vi "Illini Hyperloop GUI v2.vi"() -> ()   [LabVIEW 2015]
uses:
  <vilib>/robotics/Controls/Attitude Indicator/Attitude Indicator.xctl
  <vilib>/ErrorRing/Error Ring.xnode
panel:
  out "Attitude Indicator":cluster{"Roll":dbl, "Pitch":dbl}(xcontrol)
  out "Yaw":dbl(knob) scale=-90.0..90.0
  out "CO2 Levels":dbl format="%#.3g%%"
  out "O2 Levels":dbl format="%#.3g%%"
  out "Temperature 2":dbl(slide) scale=0.0..400.0
  out "Temp 2:":dbl format="%.2g"
  out "Temp 1:":dbl format="%.2g"
  out "Temperature 1":dbl(slide) scale=0.0..400.0
  out "Cabin Pressure":dbl format="%#.3g"
  out "Pressure":dbl(slide) scale=0.0..20.0
  out "Battery 3:":dbl format="%#.2g"
  out "Battery 2:":dbl format="%#.2g"
  out "Battery 1:":dbl format="%#.2g"
  out "Battery 3":dbl(slide) scale=0.0..100.0
  out "Battery 2":dbl(slide) scale=0.0..100.0
  out "Battery 1":dbl(slide) scale=0.0..100.0
  out "Z acceleration":dbl
  out "Y acceleration":dbl
  out "X acceleration":dbl
  out "Z velocity":dbl
  out "Y velocity":dbl
  out "X velocity":dbl
  out "Z position":dbl
  out "Y position":dbl
  out "X position":dbl
  out "Position (m)":dbl(slide) scale=0.0..2490.0
  in  "EMERGENCY STOP":bool
  out "Data out":string
  in  "Client Closed":string="The client VI closed the connection."
  in  "Functional Test 1":bool caption="Boolean"
  in  "Functional Test 2":bool caption="Boolean"
  in  "Functional Test 4":bool caption="Boolean"
  in  "Functional Test 3":bool caption="Boolean"
  out "Alarms":dbl
  out "Enum":enum16{"All Systems Nominal", "Alarm", ""}(ring)
  out "Ring":u16(ring)
  out "Velocity (m/s)":dbl(graph)
  out "Position":dbl
  out "Velocity":dbl
  out "Acceleration":dbl
  # "Illini Hyperloop"
  # "Functional Test A"
  # "Power Up"
  # "All Systems"
  # "*RESULTS DISPLAYED HERE*"
  # "Acceleration (m/s/s)"
  # "Functional Test B"
  # "Levitation"
  # "*RESULTS DISPLAYED HERE*"
  # "Functional Test C"
  # "Communication"
  # "Battery Levels (%)"
  # "Cabin Pressure (psi)"
  # "O2 Level"
  # "*RESULTS DISPLAYED HERE*"
  # "CO2 Level"
  # "Functional Test D"
  # "Internal Power"
  # "Attitude"
  # "*RESULTS DISPLAYED HERE*"
  # "Temperature (K)"
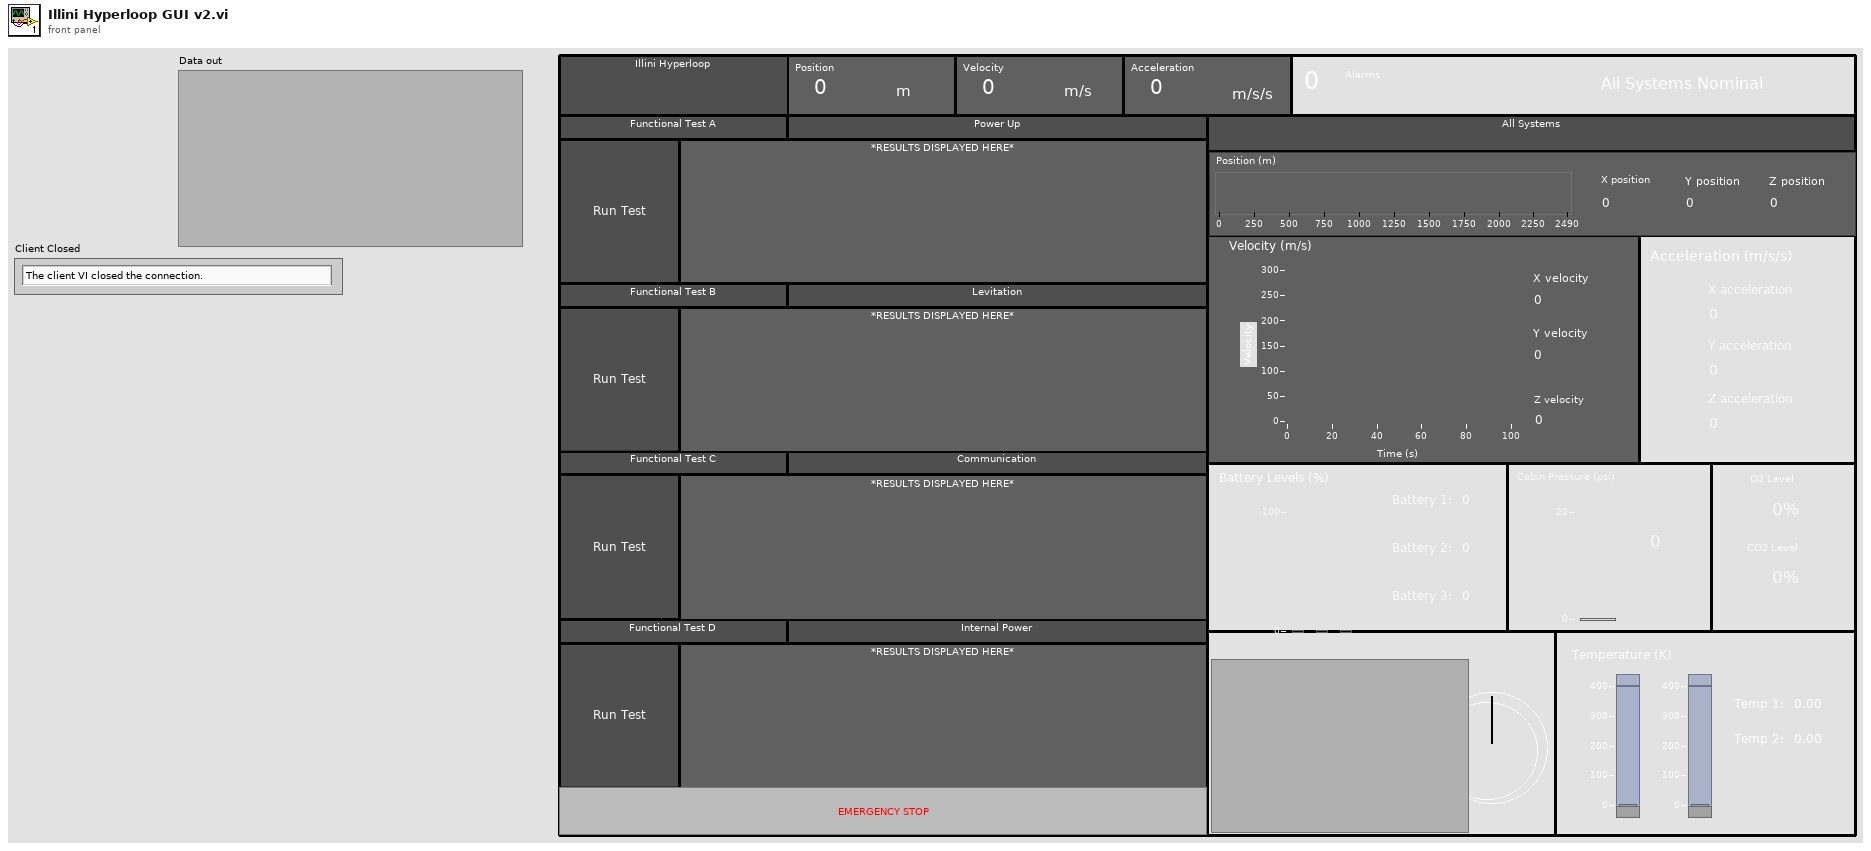
[diagram p1: front panel]
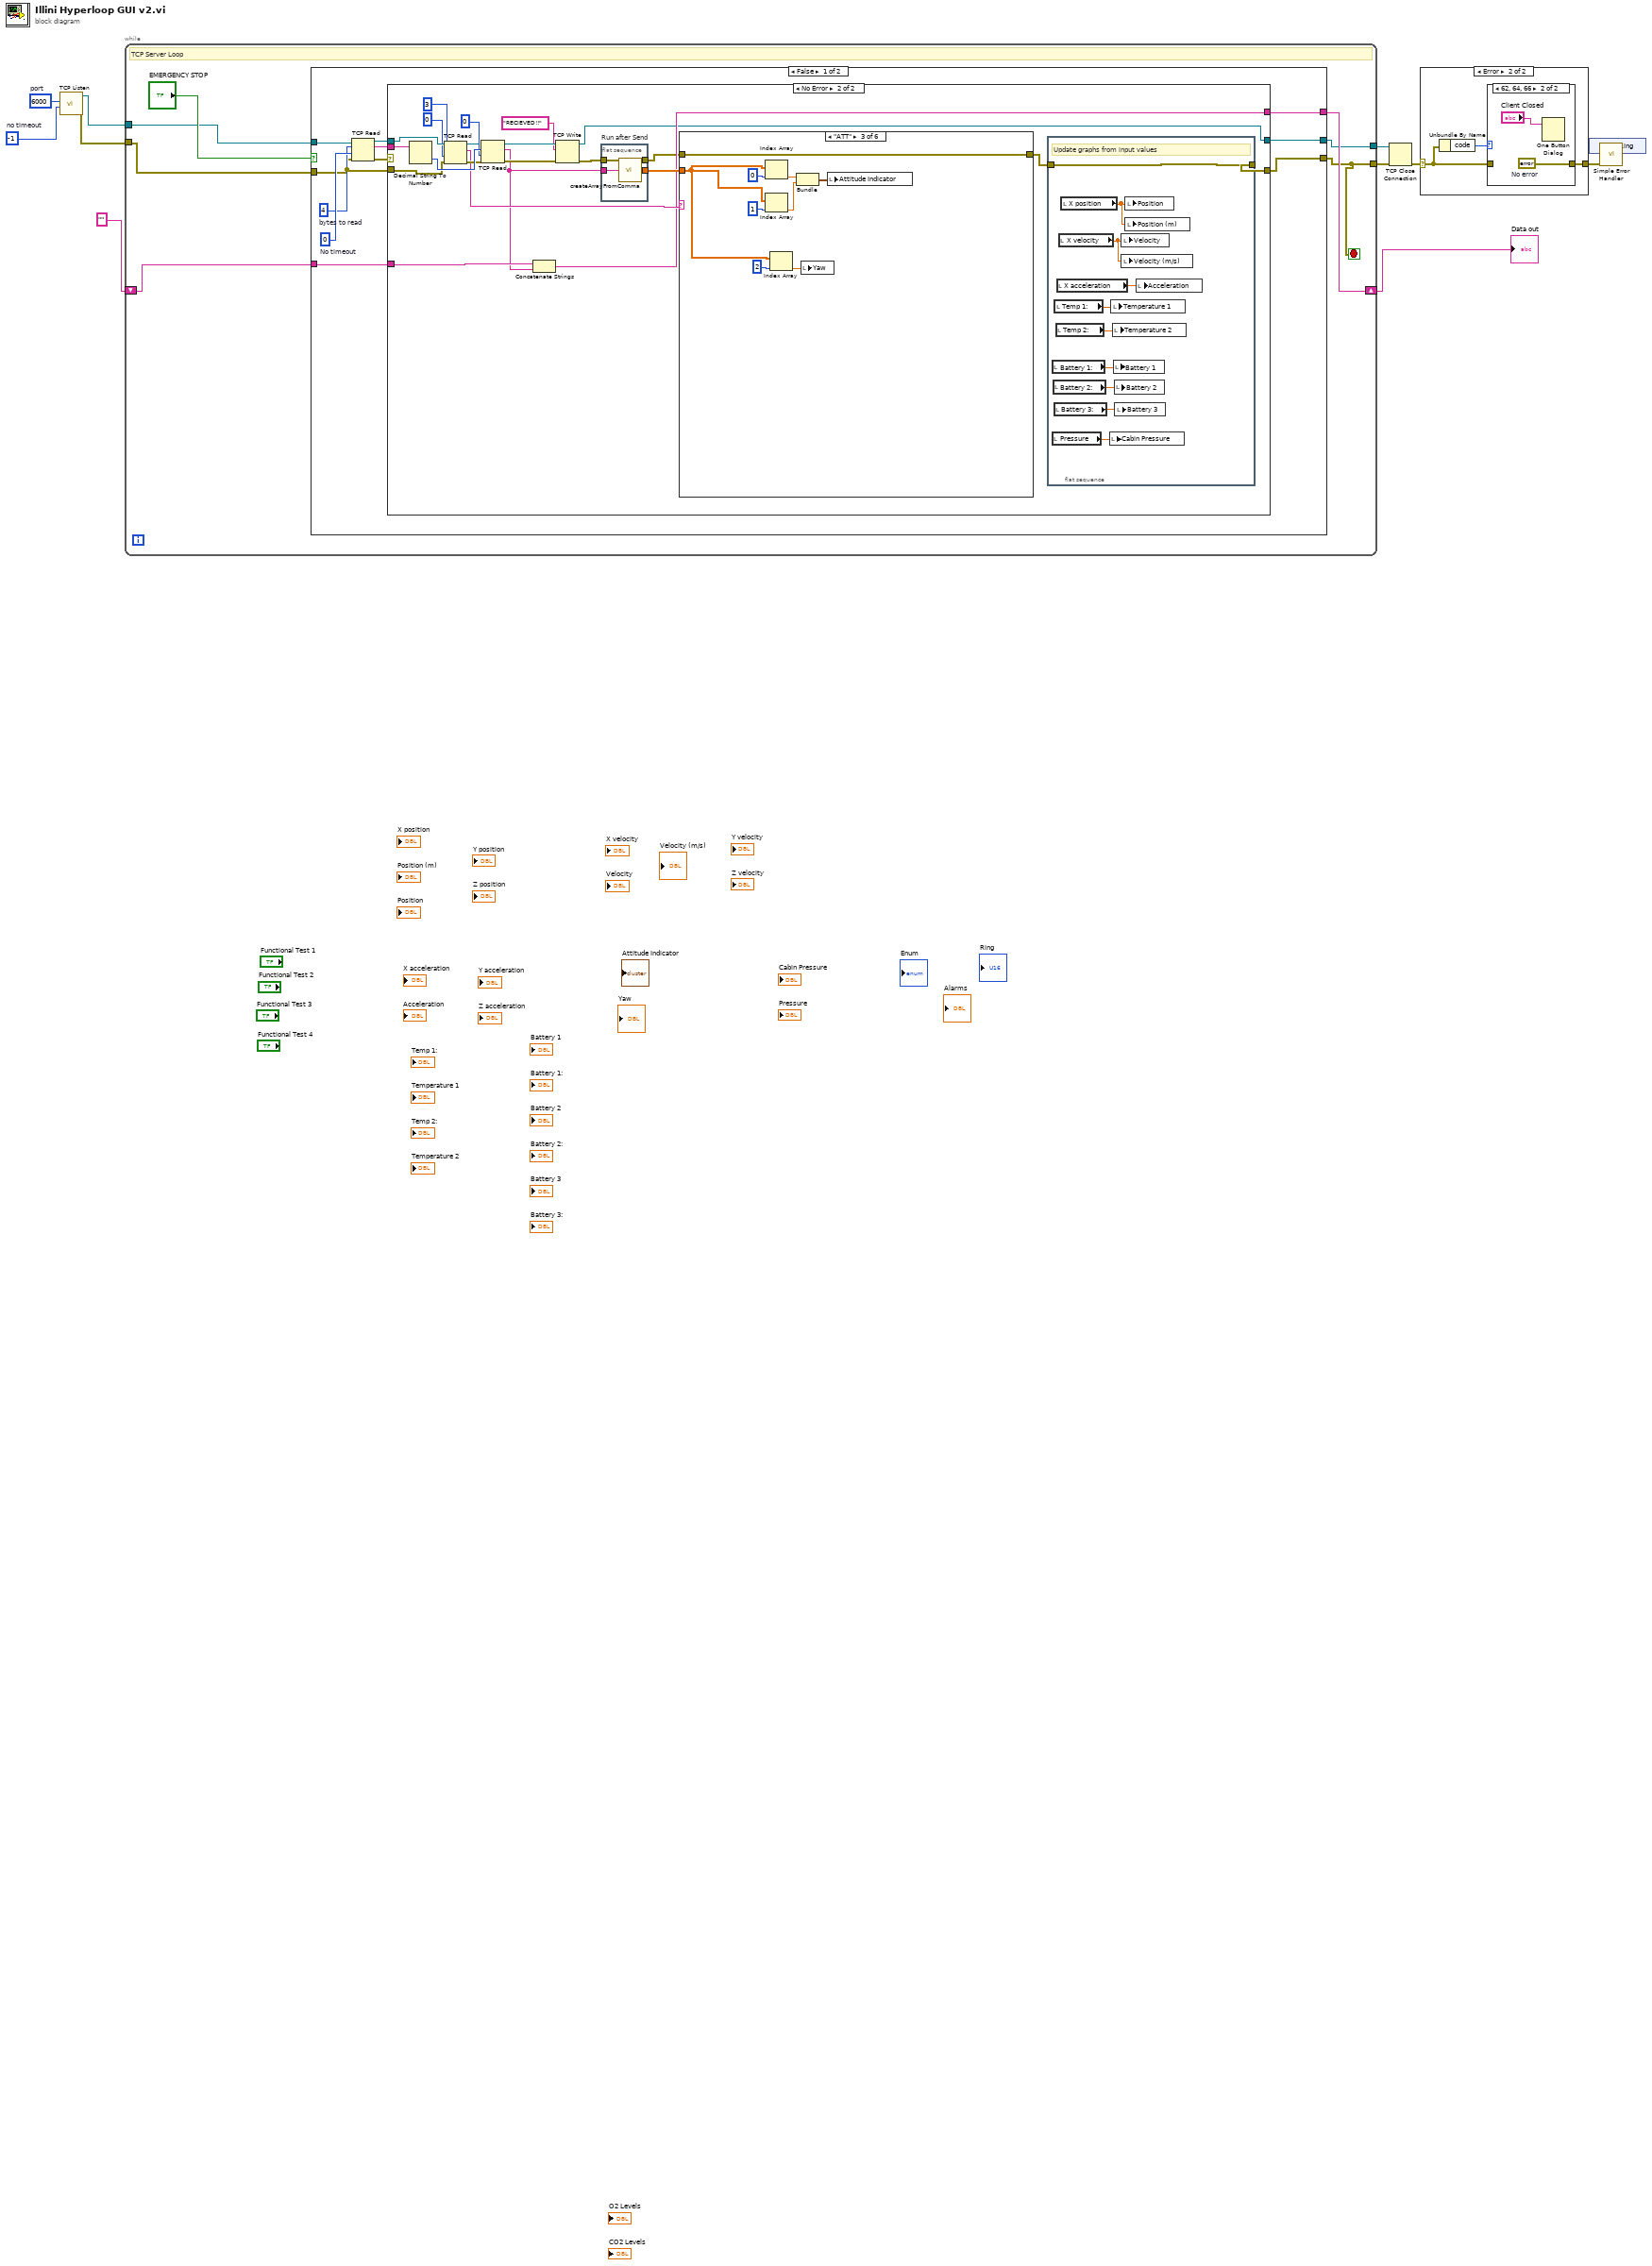
[diagram p0: block diagram]
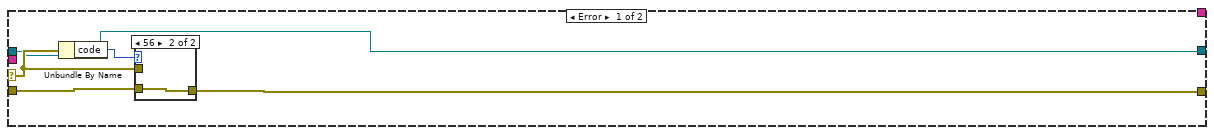
[diagram p4: hidden frame]
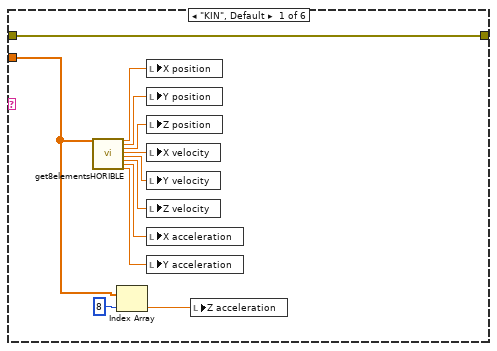
[diagram p6: hidden frame]
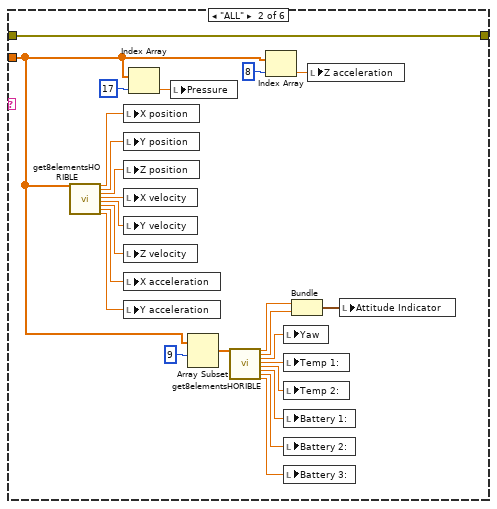
[diagram p7: hidden frame]
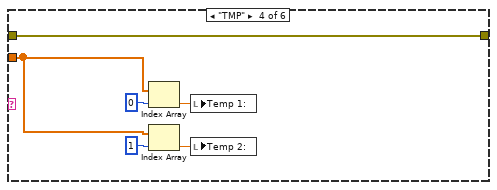
[diagram p8: hidden frame]
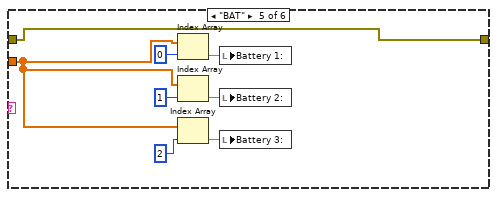
[diagram p9: hidden frame]
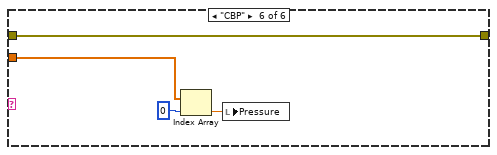
[diagram p10: hidden frame]
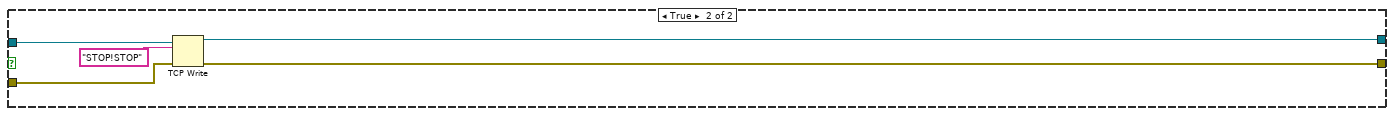
[diagram p11: hidden frame]
diagram:
  w6 = u16 6000  # port
  w7 = -1  # no timeout
  n1 = call <vilib>:"TCP Listen.vi"("timeout ms (wait forever: -1)"=w7, "port"=w6) -> ("error out"=w8:errorcluster, "connection ID"=w3:refnum<k5>)  [unwired: 5 in, 3 out]
  n2 = while {
    tunnel: w3 -> [w15]
    tunnel: w8 -> [w16]
    shift-right: [w13] -> w4
    shift-left: "" -> [w14]
    tunnel: [w12] -> w2
    tunnel: [w11] -> w1
    stop <- w11 stop-if-true
    # "TCP Server Loop"
    n3 = case shown="False" "EMERGENCY STOP" {
      tunnel: w16 -> [w26 w139]
      tunnel: w15 -> [w27 w138]
      tunnel: [w22 w137] -> w12
      tunnel: [w24 w136] -> w11
      tunnel: w14 -> [w20 _]
      tunnel: [w19 _] -> w13
      frame False {
        w28 = 4  # bytes to read
        w29 = 0  # No timeout
        n4 = TCP Read(connection ID=w27, bytes to read=w28, error in (no error)=w26, 9:w29) -> (connection ID out=w23:refnum<k5>, data out=w21:string, error out=w25:errorcluster)  [unwired: 1 in]
        n5 = case shown="No Error" w25 {
          selector: w25 -> [w32 _]
          tunnel: w26 -> [w33 w51]
          tunnel: [w31 w44] -> w24
          tunnel: w23 -> [w30 w57]
          tunnel: [w30 w43] -> w22
          tunnel: w21 -> [_ w58]
          tunnel: w20 -> [_ w47]
          tunnel: [_ w46] -> w19
          frame Error {
            n6 = Unbundle By Name(w32) -> ("code"=w34:i32)
            n7 = case shown="56" w34 {
              tunnel: w32 -> [w35 _]
              tunnel: [w35 w36] -> w31
              tunnel: w33 -> [_ w36]
              frame Default {
              }
              frame 56 {
              }
            }
          }
          frame No Error {
            n8 = Decimal String To Number(string=w58) -> (number=w54:i32)  [unwired: 2 in, 1 out]
            n9 = TCP Read(connection ID=w57, bytes to read=3, error in (no error)=w51, 9:0 ("timeout ms (25000)")) -> (connection ID out=w52:refnum<k5>, data out=w49:string, error out=w50:errorcluster)  [unwired: 1 in]
            n10 = TCP Read(connection ID=w52, bytes to read=w54, error in (no error)=w50, 9:0 ("timeout ms (25000)")) -> (connection ID out=w42:refnum<k5>, data out=w39:string, error out=w40:errorcluster)  [unwired: 1 in]
            n11 = Concatenate Strings(w47, w39) -> (w46:string)
            n12 = TCP Write(connection ID=w42, data in="RECIEVED!!", error in (no error)=w40) -> (connection ID out=w43:refnum<k5>, error out=w38:errorcluster)  [unwired: 1 in, 1 out]
            n13 = flat-sequence "Run after Send" {
              tunnel: [w61] -> w48
              tunnel: w39 -> [w60]
              tunnel: w38 -> [w59]
              tunnel: [w59] -> w37
              frame #0 {
                n14 = call "createArrayFromComma.vi"("String"=w60) -> ("Array"=w61:dbl[])
              }
            }
            n15 = case shown="\"ATT\"" w49 {
              tunnel: w48 -> [w82 w86 w114 w121 w128 w134]
              tunnel: w37 -> [w80 w84 w109 w118 w124 w132]
              tunnel: [w80 w84 w109 w118 w124 w132] -> w45
              frame "KIN", Default {
                n16 = call "get8elementsHORIBLE.vi"("Array"=w82) -> ("Numeric"=w79:dbl, "Numeric 2"=w78:dbl, "Numeric 3"=w77:dbl, "Numeric 4"=w76:dbl, "Numeric 5"=w75:dbl, "Numeric 6"=w74:dbl, "Numeric 7"=w73:dbl, "Numeric 8"=w72:dbl)  [unwired: 19 in]
                n17 = Index Array(array=w82, index=8) -> (element=w81:dbl)
                n18 = local write "X position"(w79) -> ()
                n19 = local write "Y position"(w78) -> ()
                n20 = local write "Z position"(w77) -> ()
                n21 = local write "X velocity"(w76) -> ()
                n22 = local write "Y velocity"(w75) -> ()
                n23 = local write "Z velocity"(w74) -> ()
                n24 = local write "X acceleration"(w73) -> ()
                n25 = local write "Y acceleration"(w72) -> ()
                n26 = local write "Z acceleration"(w81) -> ()
              }
              frame "ALL" {
                n27 = call "get8elementsHORIBLE.vi"("Array"=w86) -> ("Numeric"=w106:dbl, "Numeric 2"=w105:dbl, "Numeric 3"=w104:dbl, "Numeric 4"=w103:dbl, "Numeric 5"=w102:dbl, "Numeric 6"=w101:dbl, "Numeric 7"=w100:dbl, "Numeric 8"=w99:dbl)  [unwired: 19 in]
                n28 = local write "X position"(w106) -> ()
                n29 = local write "Y position"(w105) -> ()
                n30 = local write "Z position"(w104) -> ()
                n31 = local write "X velocity"(w103) -> ()
                n32 = local write "Y velocity"(w102) -> ()
                n33 = local write "Z velocity"(w101) -> ()
                n34 = local write "X acceleration"(w100) -> ()
                n35 = local write "Y acceleration"(w99) -> ()
                n36 = Index Array(array=w86, index=17) -> (element=w85:dbl)
                n37 = local write "Pressure"(w85) -> ()
                n38 = Array Subset(array=w86, index=9) -> (w96:dbl[])  [unwired: 1 in]
                n39 = call "get8elementsHORIBLE.vi"("Array"=w96) -> ("Numeric"=w95:dbl, "Numeric 2"=w94:dbl, "Numeric 3"=w93:dbl, "Numeric 4"=w92:dbl, "Numeric 5"=w91:dbl, "Numeric 6"=w90:dbl, "Numeric 7"=w89:dbl, "Numeric 8"=w88:dbl)  [unwired: 19 in]
                n40 = Index Array(array=w86, index=8) -> (element=w107:dbl)
                n41 = local write "Yaw"(w93) -> ()
                n42 = local write "Temp 1:"(w92) -> ()
                n43 = local write "Temp 2:"(w91) -> ()
                n44 = local write "Battery 1:"(w90) -> ()
                n45 = local write "Battery 2:"(w89) -> ()
                n46 = local write "Battery 3:"(w88) -> ()
                n47 = Bundle("Numeric"=w95, "Numeric 2"=w94) -> (w98:cluster{"Numeric":dbl, "Numeric 2":dbl})  [unwired: 1 in]
                n48 = local write "Z acceleration"(w107) -> ()
                n49 = local write "Attitude Indicator"(w98) -> ()
              }
              frame "ATT" {
                n50 = Index Array(array=w114, index=0) -> (element=w113:dbl)
                n51 = Index Array(array=w114, index=1) -> (element=w112:dbl)
                n52 = Index Array(array=w114, index=2) -> (element=w110:dbl)
                n53 = Bundle(w113, w112) -> (w111:cluster{dbl, dbl})  [unwired: 1 in]
                n54 = local write "Yaw"(w110) -> ()
                n55 = local write "Attitude Indicator"(w111) -> ()
              }
              frame "TMP" {
                n56 = Index Array(array=w121, index=0) -> (element=w120:dbl)
                n57 = Index Array(array=w121, index=1) -> (element=w119:dbl)
                n58 = local write "Temp 1:"(w120) -> ()
                n59 = local write "Temp 2:"(w119) -> ()
              }
              frame "BAT" {
                n60 = Index Array(array=w128, index=0) -> (element=w127:dbl)
                n61 = Index Array(array=w128, index=1) -> (element=w126:dbl)
                n62 = Index Array(array=w128, index=2) -> (element=w125:dbl)
                n63 = local write "Battery 1:"(w127) -> ()
                n64 = local write "Battery 2:"(w126) -> ()
                n65 = local write "Battery 3:"(w125) -> ()
              }
              frame "CBP" {
                n66 = Index Array(array=w134, index=0) -> (element=w133:dbl)
                n67 = local write "Pressure"(w133) -> ()
              }
            }
            n68 = flat-sequence {
              tunnel: w45 -> [w66]
              tunnel: [w66] -> w44
              frame #0 {
                # "Update graphs from input values"
                n69 = local read "Battery 1:"() -> (w65:dbl)
                n70 = local read "Pressure"() -> (w62:dbl)
                n71 = local read "Battery 2:"() -> (w64:dbl)
                n72 = local read "Battery 3:"() -> (w63:dbl)
                n73 = local read "Temp 1:"() -> (w68:dbl)
                n74 = local read "Temp 2:"() -> (w67:dbl)
                n75 = local read "X acceleration"() -> (w69:dbl)
                n76 = local read "X velocity"() -> (w70:dbl)
                n77 = local read "X position"() -> (w71:dbl)
                n78 = local write "Cabin Pressure"(w62) -> ()
                n79 = local write "Temperature 1"(w68) -> ()
                n80 = local write "Temperature 2"(w67) -> ()
                n81 = local write "Battery 1"(w65) -> ()
                n82 = local write "Battery 2"(w64) -> ()
                n83 = local write "Battery 3"(w63) -> ()
                n84 = local write "Velocity"(w70) -> ()
                n85 = local write "Velocity (m/s)"(w70) -> ()
                n86 = local write "Position"(w71) -> ()
                n87 = local write "Position (m)"(w71) -> ()
                n88 = local write "Acceleration"(w69) -> ()
              }
            }
          }
        }
      }
      frame True {
        n89 = TCP Write(connection ID=w138, data in="STOP!STOP", error in (no error)=w139) -> (connection ID out=w137:refnum<k5>, error out=w136:errorcluster)  [unwired: 1 in, 1 out]
      }
    }
    n90 = Wait (ms)(milliseconds to wait=u32 0) -> ()  [unwired: 1 out]
  }
  "Data out" <- w4
  n91 = TCP Close Connection(connection ID=w2, error in (no error)=w1) -> (error out=w10:errorcluster)  [unwired: 2 out]
  n92 = case shown="Error" w10 {
    selector: w10 -> [w141 w143]
    tunnel: [w141 w142] -> w9
    frame No Error {
    }
    frame Error {
      n93 = Unbundle By Name(w143) -> ("code"=w144:i32)
      n94 = case shown="62, 64, 66" w144 {
        tunnel: w143 -> [w145 _]
        tunnel: [w145 w147] -> w142
        frame Default {
        }
        frame 62, 64, 66 {
          w147 = errorcluster {"status"=FALSE, "code"=0, "source"=""}  # No error
          n95 = One Button Dialog(message="Client Closed") -> ()  [unwired: 1 in, 1 out]
        }
      }
    }
  }
  n96 = xnode "Error Ring"() -> ()  [unwired: 1 out]
  n97 = call <vilib>:"Simple Error Handler.vi"("error in (no error)"=w9) -> ()  [unwired: 1 in, 8 out]
